vi "Write Enabled.vi"(8 "error in (no error)":errorcluster, 10 "Enabled":bool, 11 "Robot Event in":refnum<class "Robot Event.lvclass">) -> (0 "error out":errorcluster, 3 "Robot Event out":refnum<class "Robot Event.lvclass">)   [LabVIEW 2019, in "Robot Event.lvclass"]
uses:
  Robot Event.lvclass
  Robot Event.lvclass/Robot Event.ctl
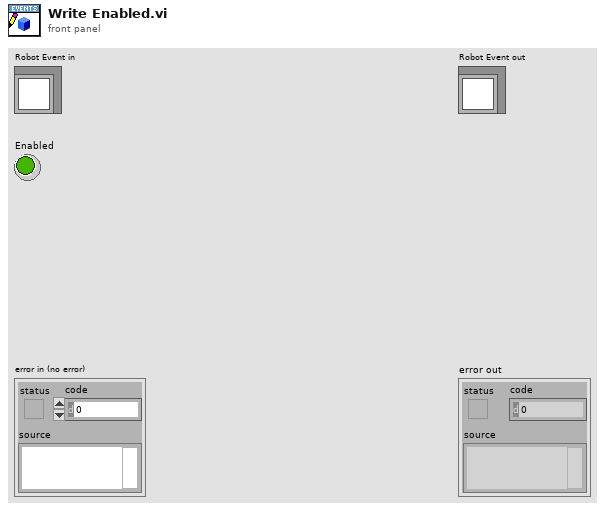
[diagram p1: front panel]
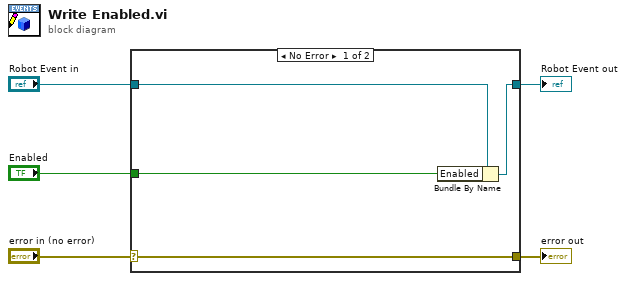
[diagram p0: block diagram]
diagram:
  n1 = case shown="No Error" "error in (no error)" {
    selector: "error in (no error)" -> [w9 w10]
    tunnel: [w9 w10] -> w4
    tunnel: [w7 w11] -> w2
    tunnel: "Robot Event in" -> [w8 w11]
    tunnel: "Enabled" -> [w6 _]
    frame No Error {
      n2 = Bundle By Name(cluster=w8, "Enabled"=w6) -> (w7:refnum<class "Robot Event.lvclass">)
    }
    frame Error {
    }
  }
  "error out" <- w4
  "Robot Event out" <- w2
